vi "creatPath.vi"(10 "string":string, 11 "Log File Base Path":path) -> (3 "appended path":path)   [LabVIEW 2020, in "Logging.lvlib"]
uses:
  Logging.lvlib
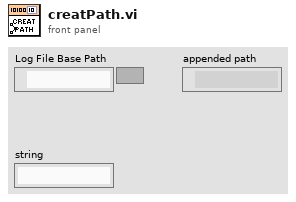
[diagram p1: front panel]
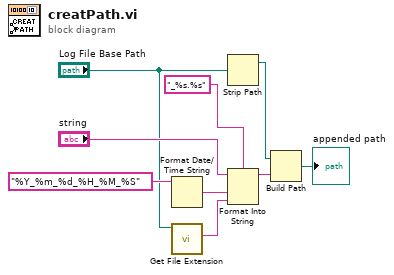
[diagram p0: block diagram]
diagram:
  n1 = Format Date/Time String(time format string (%c)="%Y_%m_%d_%H_%M_%S") -> (date/time string=w5:string)  [unwired: 2 in]
  n2 = call <vilib>:"Get File Extension.vi"("file"="Log File Base Path") -> ("lowercase file extension"=w6:string)  [unwired: 6 in, 4 out]
  n3 = Strip Path(path="Log File Base Path") -> (stripped path=w3:path)  [unwired: 1 out]
  n4 = Format Into String(format string="_%s.%s", initial string="string", w5, w6) -> (resulting string=w7:string)  [unwired: 1 in, 1 out]
  n5 = Build Path(base path=w3, name or relative path=w7) -> (appended path=→"appended path":path)
